vi "expand unbundle.vi"(8 "error in":errorcluster, 10 "Parameters to process ref in":refnum<vi>, 11 "VI Refnum":refnum<vi>) -> (0 "error out":errorcluster, 2 "unbundle ref out":refnum<vi>)   [LabVIEW 2013]
uses:
  <vilib>/Utility/traverseref.llb/TRef TravTarget.ctl
  <vilib>/Utility/traverseref.llb/VI Scripting - Traverse.lvlib
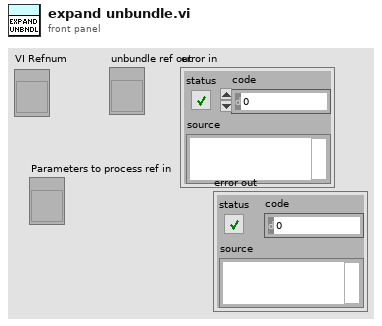
[diagram p1: front panel]
types:
  T1 = typedef "TRef TravTarget.ctl" = enum16{"FP", "BD", "Other"}
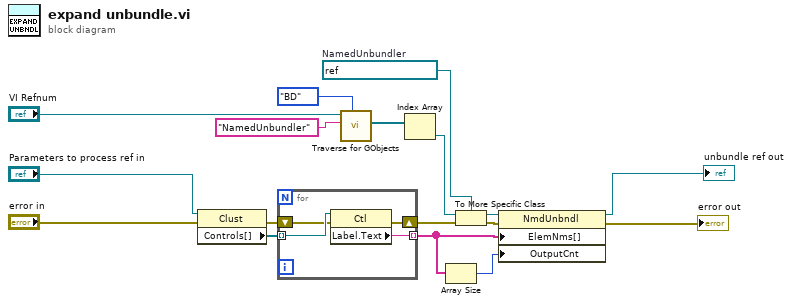
[diagram p0: block diagram]
diagram:
  w15 = refnum<vi> refnum  # NamedUnbundler
  n1 = property class="Clust"(reference="Parameters to process ref in", error in="error in") -> (error out=w13:errorcluster, "Controls[]"=w16:refnum<vi>[])  [unwired: 1 out]
  n2 = for {
    tunnel: w16 -> [w21] mode=indexing
    tunnel: [w20] -> w2 mode=indexing
    shift-right: [w18] -> w12
    shift-left: w13 -> [w19]
    n3 = property class="Ctl"(reference=w21, error in=w19) -> (error out=w18:errorcluster, "Label.Text"=w20:string)  [unwired: 1 out]
  }
  n4 = call <vilib>:"Traverse for GObjects.vi"("Traverse Target"=TRef_TravTarget."BD", "Class Name"="NamedUnbundler", "VI Refnum"="VI Refnum") -> ("References"=w7:refnum<vi>[])  [unwired: 5 in, 3 out]
  n5 = Index Array(array=w7) -> (element=w6:refnum<vi>)  [unwired: 1 in]
  n6 = Array Size(array=w2) -> (size(s)=w1:i32)
  n7 = To More Specific Class(target class=w15, reference=w6, error in=w12) -> (specific class reference=w17:refnum<vi>, error out=w11:errorcluster)
  n8 = property class="NmdUnbndl"(reference=w17, error in=w11, "ElemNms[]"=w2, "OutputCnt"=w1) -> (reference out=→"unbundle ref out":refnum<vi>, error out=→"error out":errorcluster)
